vi "AfterSpinOptions.vi"(9 "Spin at end":bool, 10 "Duration after":dbl[unit], 11 "periodic time":dbl[unit]) -> (3 "concatenated string":string)   [LabVIEW 2020]
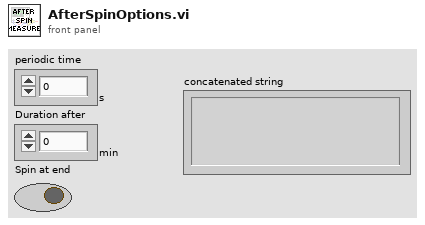
[diagram p1: front panel]
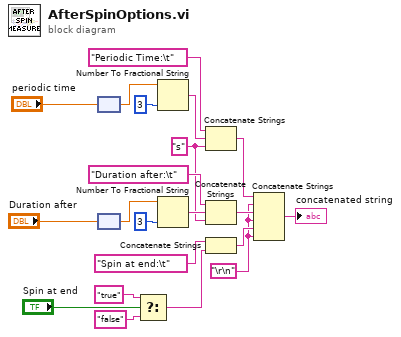
[diagram p0: block diagram]
diagram:
  w1 = "\r\n"
  w8 = "s" ("string")
  n1 = node("periodic time") -> (w18:dbl)
  n2 = node("Duration after") -> (w16:dbl)
  n3 = Select(t="true" ("string"), s="Spin at end", f="false" ("string")) -> (s? t:f=w6:string)
  n4 = Number To Fractional String(number=w18, precision (6)=i16 3) -> (F-format string=w11:string)  [unwired: 2 in]
  n5 = Number To Fractional String(number=w16, precision (6)=i16 3) -> (F-format string=w9:string)  [unwired: 2 in]
  n6 = Concatenate Strings("Periodic Time:\t" ("string"), w11, w8) -> (w4:string)
  n7 = Concatenate Strings("Duration after:\t" ("string"), w9, w8) -> (w5:string)
  n8 = Concatenate Strings("Spin at end:\t" ("string"), w6) -> (w3:string)
  n9 = Concatenate Strings(w4, w1, w5, w1, w3, w1) -> (→"concatenated string":string)
